vi "Create Bucket.vi"(6 "Access Control List":T1, 8 "error in (no error)":errorcluster, 9 "Region":T2, 10 "Name":string, 11 "AWS Credentials":T3) -> (0 "error out":errorcluster, 3 "Bucket out":refnum<class "Bucket.lvclass">)   [LabVIEW 2015, in "NI_AWS_S3.lvlib" / "Bucket.lvclass"]
doc: "This implementation of the PUT operation creates a new bucket. To create a bucket, you must register with Amazon S3 and have a valid AWS Access Key ID to authenticate requests. Anonymous requests are never allowed to create buckets. By creating the bucket, you become the bucket owner."
uses:
  Bucket.lvclass
  Core/HTTP Request/AWS Credentials.ctl
  Core/HTTP Request/Region.ctl
  ACL.ctl
  Core/HTTP Request/Request Options.ctl
  Core/HTTP Request/Name Value Pair.ctl
  Core/HTTP Request/Region handling.ctl
  Core/HTTP Request/URL formatting.ctl
  Core/HTTP Request/HTTP Request.lvclass/HTTP Request.ctl
  Bucket.lvclass/Bucket.ctl
  Core/HTTP Request/Write Credentials.vi
  Core/HTTP Request/Write Region.vi
  Core/HTTP Request/Write Service.vi
  Write Name.vi
  Core/HTTP Request/Write Verify Server.vi
  Core/HTTP Request/HTTP Request.lvclass
  NI_AWS_S3.lvlib
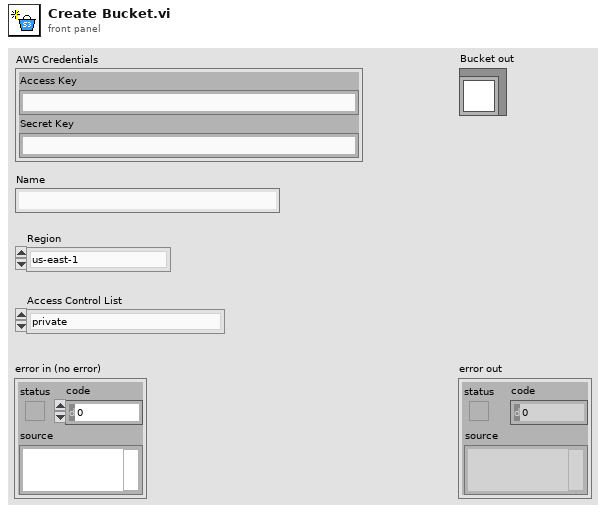
[diagram p1: front panel]
types:
  T1 = typedef "NI_AWS_S3.lvlib/ACL.ctl" = enum16{"private", "public-read", "public-read-write", "aws-exec-read", "authenticated-read", "bucket-owner-read", "bucket-owner-full-control"}
  T2 = typedef "NI_AWS_Core.lvlib/HTTP Request.lvclass/Region.ctl" = enum16{"us-east-1", "us-east-2", "us-west-1", "us-west-2", "ap-northeast-1", "ap-northeast-2", "ap-southeast-1", "ap-southeast-2", "ca-central-1", "eu-central-1", "eu-west-1", "eu-west-2", "sa-east-1"}
  T3 = typedef "NI_AWS_Core.lvlib/HTTP Request.lvclass/AWS Credentials.ctl" = cluster{"Access Key":string, "Secret Key":string}
  T4 = typedef "NI_AWS_Core.lvlib/HTTP Request.lvclass/Region handling.ctl" = enum16{"use region everywhere", "use region (authentication only)", "use region (URL only)", "ignore region everwhere"}
  T5 = typedef "NI_AWS_Core.lvlib/HTTP Request.lvclass/Request Options.ctl" = cluster{"request headers":T6[], "request parameters":T6[], "request body":string, "region handling":T4, "URL formatting":T7}
  T6 = typedef "NI_AWS_Core.lvlib/HTTP Request.lvclass/Name Value Pair.ctl" = cluster{"name":string, "value":string}
  T7 = typedef "NI_AWS_Core.lvlib/HTTP Request.lvclass/URL formatting.ctl" = enum16{"region-", "region."}
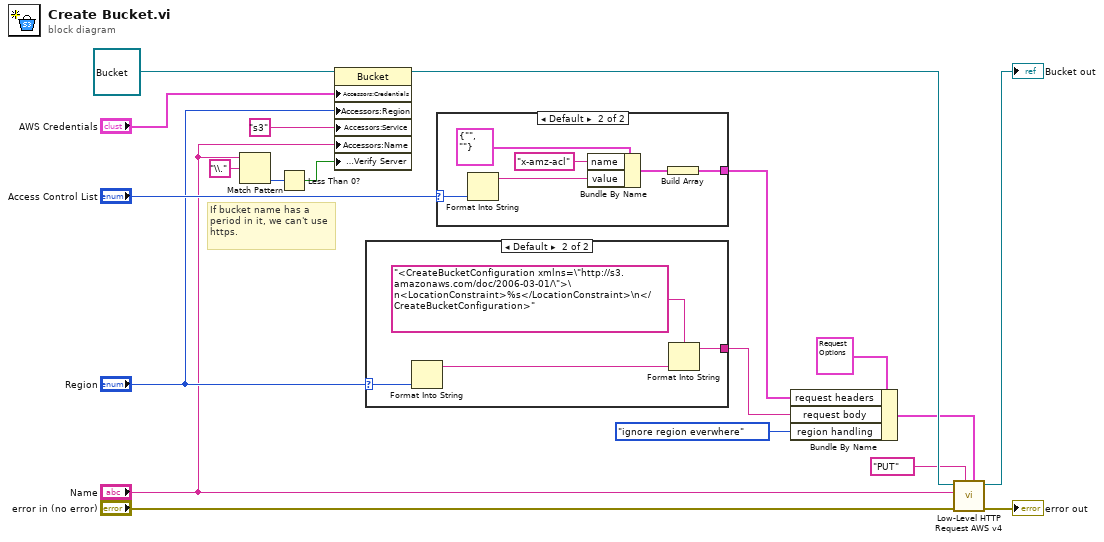
[diagram p0: block diagram]
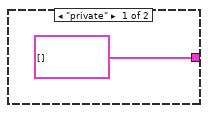
[diagram p3: hidden frame]
diagram:
  # "If bucket name has a period in it, we can't use https."
  n1 = Match Pattern(string="Name", regular expression="\\.") -> (offset past match=w3:i32)  [unwired: 1 in, 3 out]
  n2 = Less Than 0?(x=w3) -> (x < 0?=w1:bool)
  n3 = property class="Bucket"(reference=refnum<class "Bucket.lvclass"> refnum ("NI_AWS_S3.lvlib:Bucket.lvclass"), "Accessors:Credentials"="AWS Credentials", "Accessors:Region"="Region", "Accessors:Service"="s3" ("Service"), "Accessors:Name"="Name", "Accessors:Verify Server"=w1) -> (reference out=w8:refnum<class "Bucket.lvclass">)  [unwired: 1 in, 1 out]
  n4 = case shown="Default" "Region" {
    selector: "Region" -> [_ w23]
    tunnel: [_ w20] -> w9
    frame "us-east-1" {
    }
    frame Default {
      n5 = Format Into String(w23) -> (resulting string=w21:string)  [unwired: 3 in, 1 out]
      n6 = Format Into String(format string="<CreateBucketConfiguration xmlns=\"http://s3.amazonaws.com/doc/2006-03-01/\">\n<LocationConstraint>%s</LocationConstraint>\n</CreateBucketConfiguration>", w21) -> (resulting string=w20:string)  [unwired: 2 in, 1 out]
    }
  }
  n7 = case shown="Default" "Access Control List" {
    selector: "Access Control List" -> [_ w26]
    tunnel: [T6[] [] w27] -> w11
    frame "private" {
    }
    frame Default {
      n8 = Format Into String(w26) -> (resulting string=w25:string)  [unwired: 3 in, 1 out]
      n9 = Bundle By Name(cluster=T6 {"name"="", "value"=""} ("Name Value Pair"), "name"="x-amz-acl" ("Header"), "value"=w25) -> (w28:T6)
      n10 = Build Array(w28) -> (w27:T6[])
    }
  }
  n11 = Bundle By Name(cluster=T5 {"request headers"=[], "request parameters"=[], "request body"="", "region handling"=enum."use region everywhere", "URL formatting"=enum."region."} ("Request Options"), "request headers"=w11, "request body"=w9, "region handling"=Region_handling."ignore region everwhere") -> (w6:T5)
  n12 = call "Low-Level HTTP Request AWS v4.vi"("Request Options"=w6, "HTTP-Verb"="PUT", "error in (no error)"="error in (no error)", "URL Prefix"="Name", "AWS Core in"=w8) -> ("error out"=→"error out":errorcluster, "AWS Core out"=→"Bucket out":refnum<class "Bucket.lvclass">)  [unwired: 3 in, 2 out]
